vi "3rd_FilePaths.vi"() -> (0 "AppFiles on RIO":string="files/c/ni-rt/startup/AppKeyFiles", 2 "Device Folder":path, 3 "AppKey Files":path)   [LabVIEW 2016]
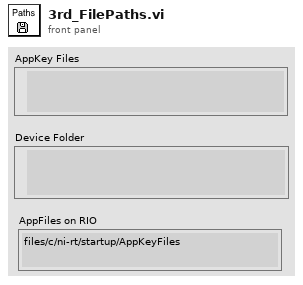
[diagram p1: front panel]
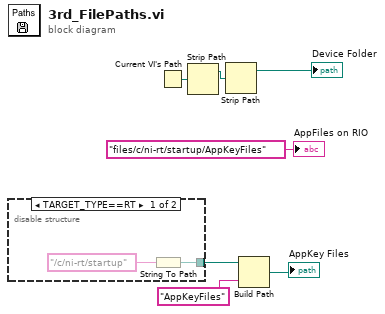
[diagram p0: block diagram]
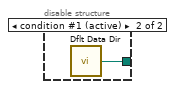
[diagram p2: hidden frame]
diagram:
  n1 = disable-structure shown="TARGET_TYPE==RT" {
    disable-tunnel: [w9 w10] -> w6
    frame condition #0 {
      n2 = String To Path(string="/c/ni-rt/startup" ("relative uri")) -> (path=w9:path)
    }
    frame condition #1 (active) {
      n3 = call <vilib>:"Dflt Data Dir.vi"() -> ("App:Default Data Directory"=w10:path)
    }
  }
  n4 = Current VI's Path() -> (path=w3:path)
  n5 = Strip Path(path=w3) -> (stripped path=w4:path)  [unwired: 1 out]
  n6 = Strip Path(path=w4) -> (stripped path=→"Device Folder":path)  [unwired: 1 out]
  n7 = Build Path(base path=w6, name or relative path="AppKeyFiles") -> (appended path=→"AppKey Files":path)
  "AppFiles on RIO" <- "files/c/ni-rt/startup/AppKeyFiles" ("relative uri")
